vi "Data-log-ins-data.vi"(7 "Scheduler State":T2, 9 "Plant 2 State":dbl[](array[numeric]), 10 "Plant 1 State":dbl[](array[numeric]), 11 "Data cluster in":cluster{"Plant 2":T1, "Plant 1":T1}) -> (3 "Data cluster out":cluster{"Plant 2":T1, "Plant 1":T1})   [LabVIEW 2016]
uses:
  Sched_state.ctl
  Plant_info.ctl
  Plant-data.ctl
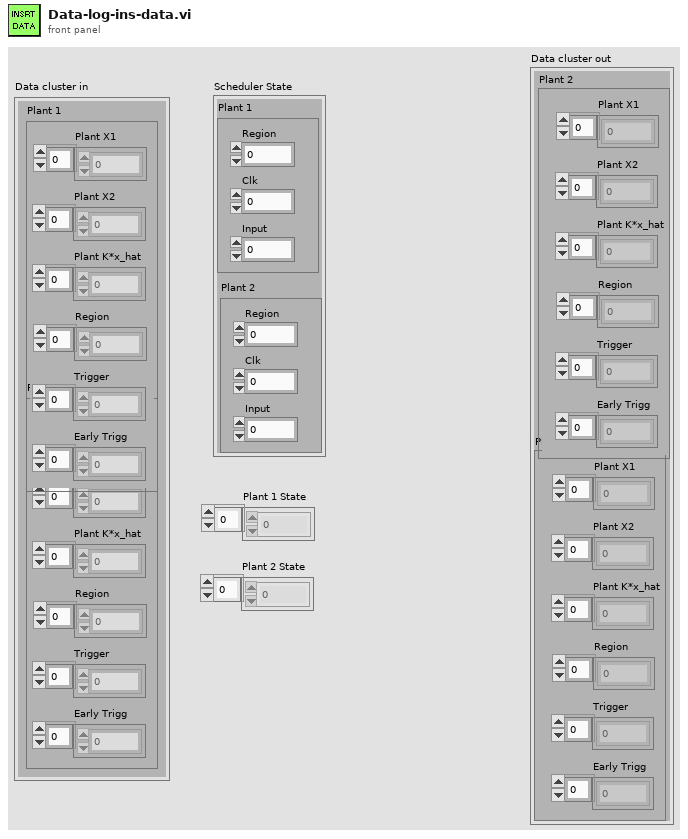
[diagram p1: front panel]
types:
  T1 = typedef "Plant-data.ctl" = cluster{"Plant X1 ":dbl[], "Plant X2":dbl[], "Plant K*x_hat":dbl[], "Region":i32[], "Trigger":i32[], "Early Trigg":i32[]}
  T2 = typedef "Sched_state.ctl" = cluster{"Plant 1":T3, "Plant 2":T3}
  T3 = typedef "Plant_info.ctl" = cluster{"Clk":dbl, "Region":dbl, "Input":dbl}
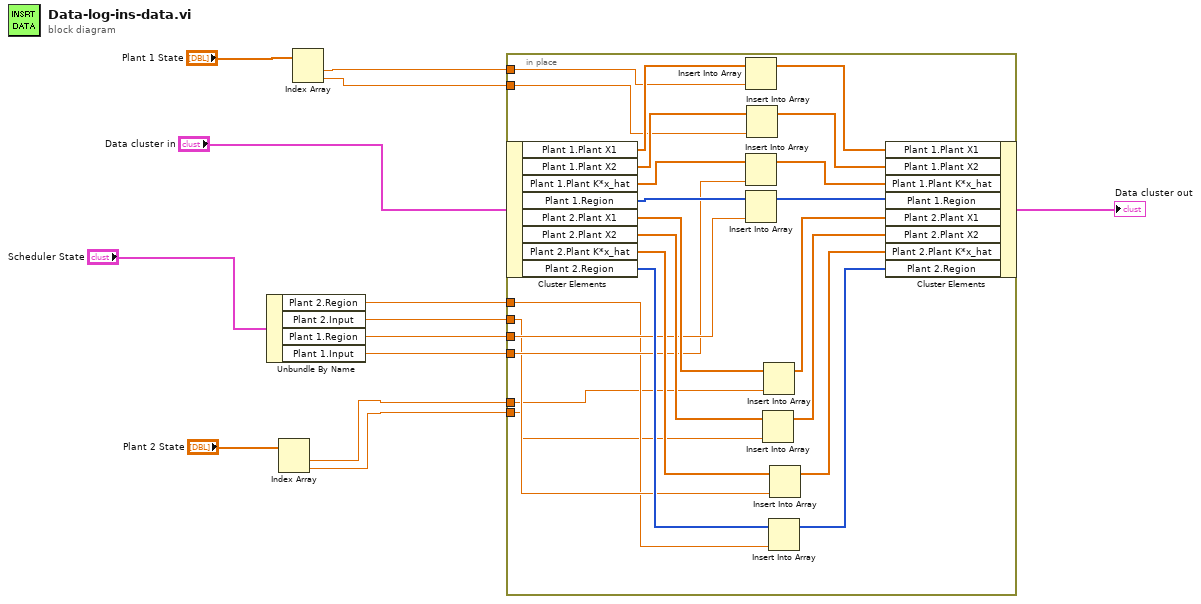
[diagram p0: block diagram]
diagram:
  n1 = Unbundle By Name("Scheduler State") -> ("Plant 2.Region"=w11:dbl, "Plant 2.Input"=w10:dbl, "Plant 1.Region"=w9:dbl, "Plant 1.Input"=w8:dbl)
  n2 = Index Array(array="Plant 2 State") -> (element #1=w3:dbl, element #2=w2:dbl)  [unwired: 2 in]
  n3 = Index Array(array="Plant 1 State") -> (element #1=w6:dbl, element #2=w5:dbl)  [unwired: 2 in]
  n4 = in-place {
    in-place-border: w11 -> [w24]
    in-place-border: w10 -> [w25]
    in-place-border: w9 -> [w29]
    in-place-border: w8 -> [w28]
    in-place-border: w6 -> [w27]
    in-place-border: w5 -> [w26]
    in-place-border: w3 -> [w23]
    in-place-border: w2 -> [w22]
    n5 = in-place-cluster #1("Data cluster in") -> ("Plant 1.Plant X1"=w37:dbl[], "Plant 1.Plant X2"=w36:dbl[], "Plant 1.Plant K*x_hat"=w35:dbl[], "Plant 1.Region"=w34:i32[], "Plant 2.Plant X1"=w33:dbl[], "Plant 2.Plant X2"=w32:dbl[], "Plant 2.Plant K*x_hat"=w31:dbl[], "Plant 2.Region"=w30:i32[])
    n6 = Insert Into Array(array=w37, new element=w27) -> (w21:dbl[])  [unwired: 1 in]
    n7 = Insert Into Array(array=w35, new element=w28) -> (w19:dbl[])  [unwired: 1 in]
    n8 = Insert Into Array(array=w34, new element=w29) -> (w18:i32[])  [unwired: 1 in]
    n9 = Insert Into Array(array=w36, new element=w26) -> (w20:dbl[])  [unwired: 1 in]
    n10 = Insert Into Array(array=w32, new element=w22) -> (w16:dbl[])  [unwired: 1 in]
    n11 = Insert Into Array(array=w33, new element=w23) -> (w17:dbl[])  [unwired: 1 in]
    n12 = Insert Into Array(array=w30, new element=w24) -> (w14:i32[])  [unwired: 1 in]
    n13 = Insert Into Array(array=w31, new element=w25) -> (w15:dbl[])  [unwired: 1 in]
    n14 = in-place-cluster #1("Plant 1.Plant X1"=w21, "Plant 1.Plant X2"=w20, "Plant 1.Plant K*x_hat"=w19, "Plant 1.Region"=w18, "Plant 2.Plant X1"=w17, "Plant 2.Plant X2"=w16, "Plant 2.Plant K*x_hat"=w15, "Plant 2.Region"=w14) -> (→"Data cluster out":cluster{"Plant 2":T1, "Plant 1":T1})
  }
